vi "run_chatcompletion.vi"(0 "chatcompletion_llm_interface in":refnum<class "llm_ollama_chatmodels.lvclass">, 5 "Messages":refnum<class "abstract_message_base.lvclass">[](array[class]), 11 "error in (no error)":errorcluster) -> (4 "chatcompletion_llm_interface out":refnum<class "llm_ollama_chatmodels.lvclass">, 6 "chat response":string, 15 "error out":errorcluster)   [LabVIEW 2020, in "llm_ollama_chatmodels.lvclass"]
uses:
  llm_ollama_chatmodels.lvclass
  abstract_message_base/abstract_message_base.lvclass
  <vilib>/httpClient/POSTBuffer.vi
  llm_ollama_chatmodels.lvclass/llm_ollama_chatmodels.ctl
  <vilib>/httpClient/LabVIEWHTTPClient.lvlib
panel:
  out "body":string
  out "headers":string
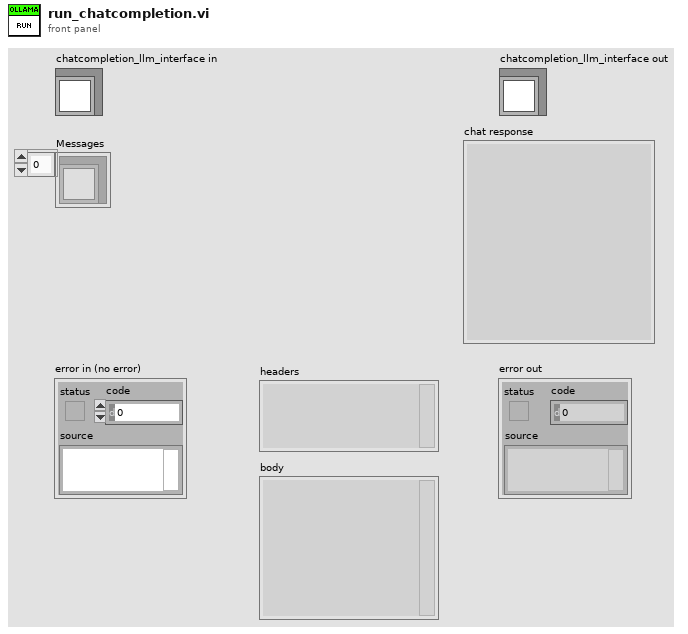
[diagram p1: front panel]
types:
  T1 = typedef "LabVIEWHTTPClient.lvlib/ClientHandle.ctl" = refnum<k1>
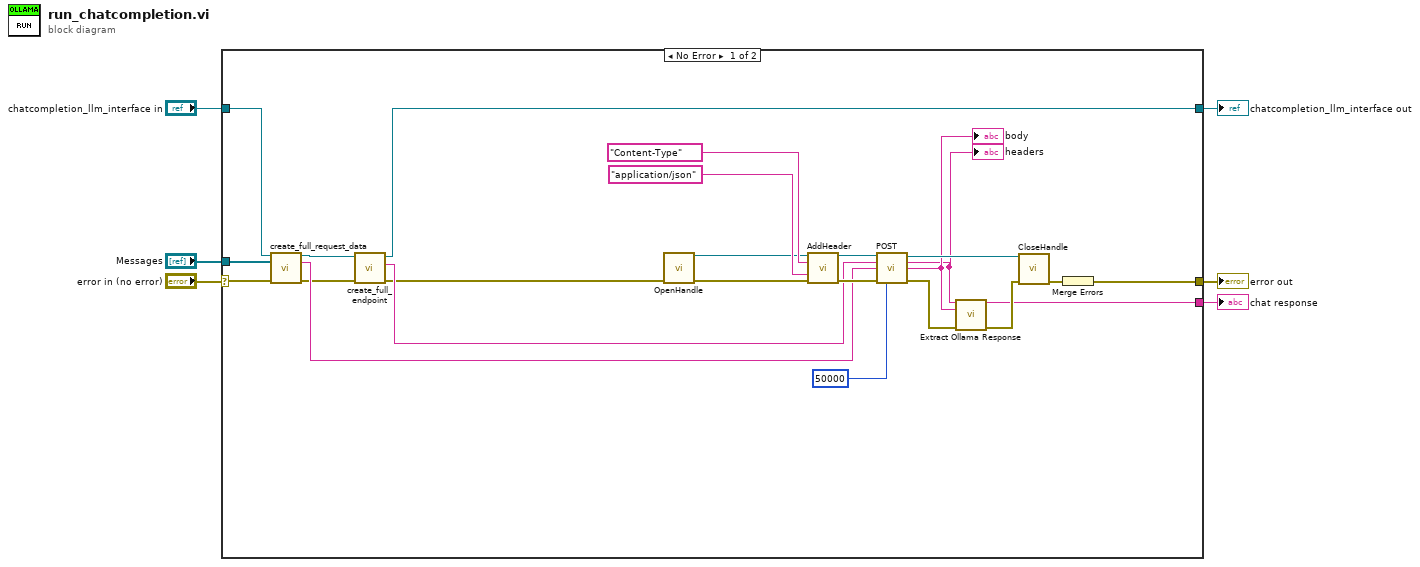
[diagram p0: block diagram]
diagram:
  n1 = case shown="No Error" "error in (no error)" {
    selector: "error in (no error)" -> [w14 w32]
    tunnel: [w17 w32] -> w5
    tunnel: "chatcompletion_llm_interface in" -> [w16 w31]
    tunnel: [w8 w31] -> w3
    tunnel: [w20 _] -> w2
    tunnel: "Messages" -> [w15 _]
    frame No Error {
      n2 = call-dynamic "create_full_request_data.vi"("llm_openai_chatmodels in"=w16, "Messages"=w15, "error in (no error)"=w14) -> ("llm_openai_chatmodels out"=w12:refnum<class "llm_ollama_chatmodels.lvclass">, "Request Data"=w13:string, "error out"=w11:errorcluster)  [unwired: 10 in]
      n3 = call-dynamic "create_full_endpoint.vi"("error in (no error)"=w11, "llm_openai_chatmodels in"=w12) -> ("error out"=w9:errorcluster, "endpoint"=w10:string, "llm_openai_chatmodels out"=w8:refnum<class "llm_ollama_chatmodels.lvclass">)  [unwired: 7 in]
      n4 = call <vilib>:"OpenHandle.vi"("error in (no error)"=w9) -> ("client handle out"=w28:T1, "error out"=w26:errorcluster)  [unwired: 13 in]
      n5 = call <vilib>:"AddHeader.vi"("client handle"=w28, "header"="Content-Type", "value"="application/json", "error in (no error)"=w26) -> ("client handle out"=w27:T1, "error out"=w25:errorcluster)  [unwired: 10 in]
      n6 = call-poly <vilib>:"POST.vi"("client handle"=w27, "url"=w10, "buffer"=w13, "error in (no error)"=w25, "timeout (10000)"=50000) -> ("client handle out"=w23:T1, "headers"=w18:string, "body"=w19:string, "error out"=w22:errorcluster)  [unwired: 7 in]
      "headers" <- w18
      "body" <- w19
      n7 = call "Extract Ollama Response.vi"("headers"=w18, "body"=w19, "error in"=w22) -> ("value"=w20:string, "error out"=w21:errorcluster)  [unwired: 11 in]
      n8 = call <vilib>:"CloseHandle.vi"("client handle"=w23, "error in (no error)"=w21) -> ("error out"=w24:errorcluster)  [unwired: 13 in]
      n9 = Merge Errors(w24) -> (w17:errorcluster)
    }
    frame Error {
    }
  }
  "error out" <- w5
  "chatcompletion_llm_interface out" <- w3
  "chat response" <- w2
